vi "Prepare Request.vi"(11 "Request in":refnum<class "Request.lvclass">) -> (3 "Request out":refnum<class "Request.lvclass">)   [LabVIEW 2020, in "OAuth2.lvlib" / "Request.lvclass"]
uses:
  Request.lvclass
  OAuth2.lvlib
  lv-web-crypto/lv-crypto/Crypto/Crypto.lvlib
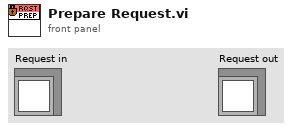
[diagram p1: front panel]
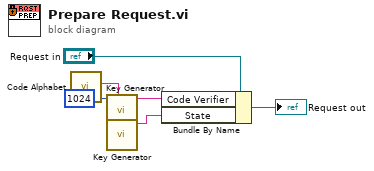
[diagram p0: block diagram]
diagram:
  n1 = call "Code Alphabet.vi"() -> ("Code Alphabet"=w5:string)  [unwired: 11 in]
  n2 = call "Key Generator.vi"("Alphabet (Default)"=w5, "Bits (256)"=1024) -> ("Key"=w4:string)  [unwired: 8 in, 1 out]
  n3 = call "Key Generator.vi"("Alphabet (Default)"=w5) -> ("Key"=w3:string)  [unwired: 9 in, 1 out]
  n4 = Bundle By Name(cluster="Request in", "Code Verifier"=w4, "State"=w3) -> (→"Request out":refnum<class "Request.lvclass">)
